vi "_Raise Save As UI Showing.vi"(4 "WebView2.lvlib:WebView2 Control.lvclass":refnum<class "WebView2 Control.lvclass">, 5 "Event Data":cluster{"sender":refnum<k24>, "e":refnum<k24>}, 6 "Control Ref":refnum<k24>, 7 "Event Common Data":T1) -> ()   [LabVIEW 2025, in "WebView2.lvlib" / "WebView2 Control.lvclass"]
uses:
  WebView2 Control.lvclass
  WebView2 Control.lvclass/WebView2 Control.ctl
  E:/Labview/LV 2023/PPL/PPL Builder/Libs/LV-WebView2/Source/Libs/Microsoft.Web.WebView2.Core.dll
  Libs/Microsoft.Web.WebView2.Core.dll
  WebView2 Event Filter Interface/WebView2 Event Filter Interface.lvclass
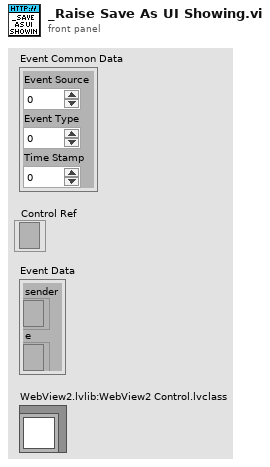
[diagram p1: front panel]
types:
  T1 = cluster{"Event Source":i32, "Event Type":u32, "Time Stamp":u32}
  T2 = cluster{"AllowReplace":bool, "Cancel":bool, "Kind":i32, "SaveAsFilePath":string, "SuppressDefaultDialog":bool}
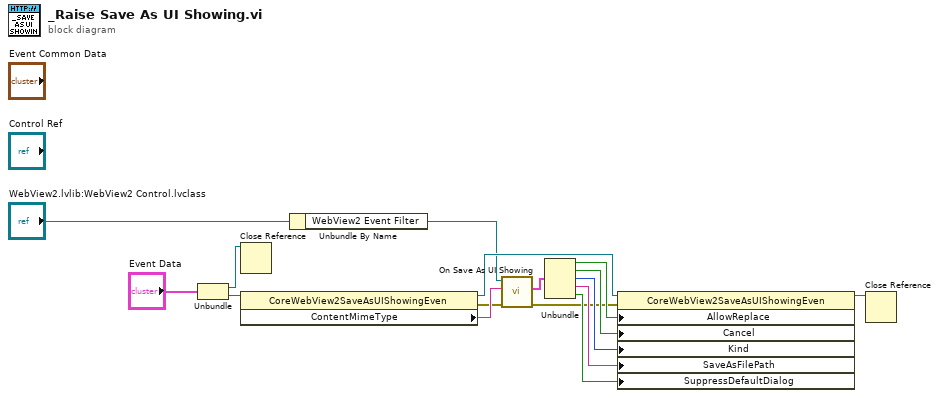
[diagram p0: block diagram]
diagram:
  n1 = Unbundle("Event Data") -> ("sender"=w15:refnum<k24>, "e"=w14:refnum<k24>)
  n2 = Close Reference(reference=w15) -> ()  [unwired: 1 in, 1 out]
  n3 = property class="CoreWebView2SaveAsUIShowingEven"(reference=w14) -> (reference out=w13:refnum<k24>, error out=w3:errorcluster, "ContentMimeType"=w10:string)  [unwired: 1 in]
  n4 = Unbundle By Name("WebView2.lvlib:WebView2 Control.lvclass") -> ("WebView2 Event Filter"=w11:refnum<class "WebView2 Event Filter Interface.lvclass">)
  n5 = call-dynamic "On Save As UI Showing.vi"("error in (no error)"=w3, "ContentMimeType"=w10, "WebView2 Event Filter Interface in"=w11) -> ("error out"=w2:errorcluster, "Response"=w9:T2)  [unwired: 7 in]
  n6 = Unbundle(w9) -> ("AllowReplace"=w8:bool, "Cancel"=w7:bool, "Kind"=w6:i32, "SaveAsFilePath"=w5:string, "SuppressDefaultDialog"=w4:bool)
  n7 = property class="CoreWebView2SaveAsUIShowingEven"(reference=w13, error in=w2, "AllowReplace"=w8, "Cancel"=w7, "Kind"=w6, "SaveAsFilePath"=w5, "SuppressDefaultDialog"=w4) -> (reference out=w1:refnum<k24>)  [unwired: 1 out]
  n8 = Close Reference(reference=w1) -> ()  [unwired: 1 in, 1 out]
